vi "Configure RT Noise.vi"(0 "VISA resource name":refnum<visa-resource-name>, 1 "Enable Noise (F:Disable)":bool, 5 "Modulation Format (1: Dual Modulation)":u16(ring)=1 items=["Dual Modulation"=1, "Dual ARB"=2, "Multitone"=3, "Two-tone"=6], 7 "Carrier Bandwidth (1 Hz)":dbl=1.0, 9 "Noise Bandwidth (1 Hz)":dbl=1.0, 11 "error in (no error)":errorcluster, 12 "Noise Bandwidth Factor (1)":u16(ring)=1 items=["1"=1, "2"=2], 13 "Noise Ratio (0 dB)":dbl) -> (4 "VISA resource name out":refnum<visa-resource-name>, 15 "error out":errorcluster)   [LabVIEW 2009, in "Agilent PSG MXG Series.lvlib"]
doc: "Configures real-time additive white gaussian noise (AWGN) added to the carrier.\n\n<B>Notes:</B>\n(1) This VI is valid only in E8267D, N5182A.\n\n(2) For E8267D, this VI is valid only when the instrument installs <B>Option 601</B> or <B>Option 602</B> (Internal baseband generator), and <B>Option 403</B> (Calibrated noise, AWGN).\n\n(3) For N5182A, this VI is valid only when the instrument installs <B>Option 403</B> (Calibrated noise, AWGN)."
uses:
  Agilent PSG MXG Series.lvlib
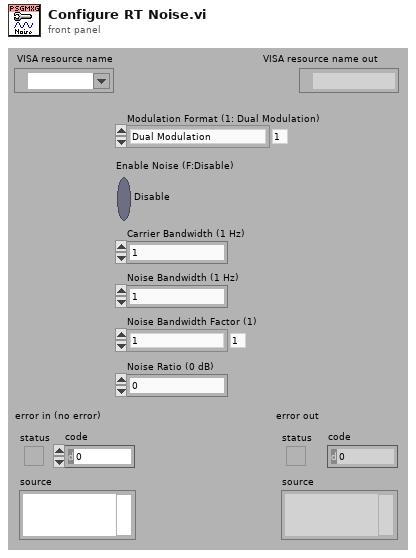
[diagram p1: front panel]
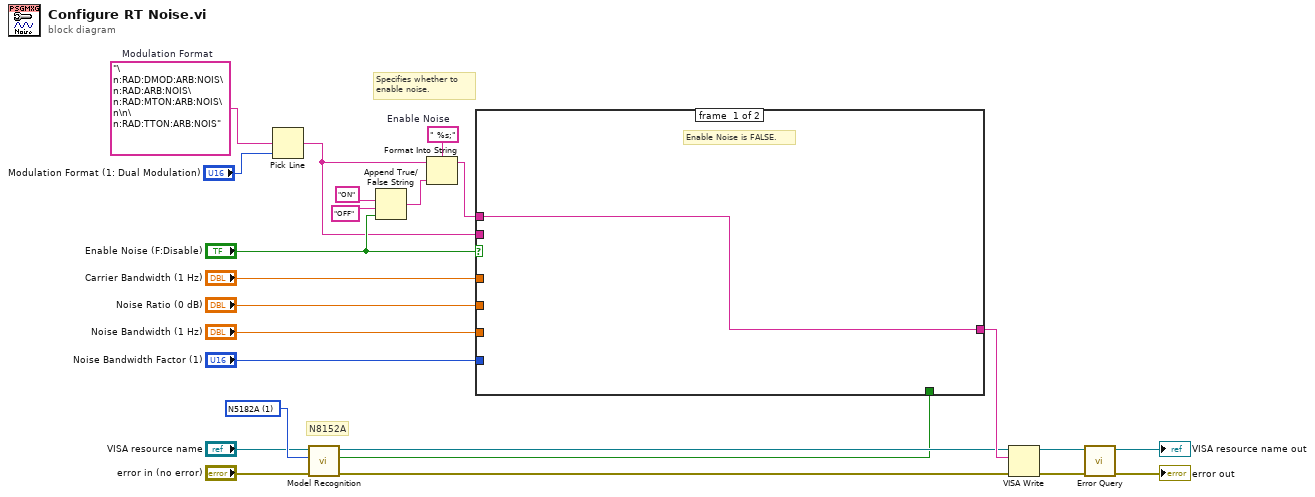
[diagram p0: block diagram]
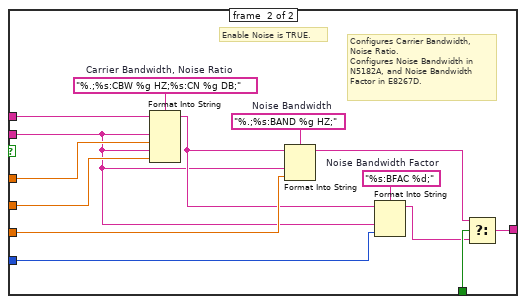
[diagram p2: hidden frame]
diagram:
  w8 = u16 1 items=["N5181A"=0, "N5182A"=1, "E8241A"=5, "E8244A"=6, "E8251A"=7, "E8254A"=8, "E8247C"=10, "E8257C"=11, "E8267C"=12, "E8257D"=15, "E8267D"=16] ("Model Type (0: N5181A)")
  w22 = " %s;"  # Enable Noise
  w24 = "\n:RAD:DMOD:ARB:NOIS\n:RAD:ARB:NOIS\n:RAD:MTON:ARB:NOIS\n\n\n:RAD:TTON:ARB:NOIS"  # Modulation Format
  # "Specifies whether to\nenable noise."
  # "N8152A"
  n1 = Pick Line(multi-line string=w24, line index="Modulation Format (1: Dual Modulation)") -> (output string=w16:string)  [unwired: 1 out]
  n2 = call "Model Recognition.vi"("error in (no error)"="error in (no error)", "Model Type (0: N5181A)"=w8, "VISA resource name"="VISA resource name") -> ("error out"=w6:errorcluster, "Is Model Correct"=w5:bool, "VISA resource name out"=w7:refnum<visa-resource-name>)  [unwired: 6 out]
  n3 = Append True/False String(1:"Enable Noise (F:Disable)", 2:"OFF" ("false string"), 3:"ON" ("true string")) -> (0:w21:string)  [unwired: 1 out]
  n4 = Format Into String(format string=w22, initial string=w16, w21) -> (resulting string=w17:string)  [unwired: 1 in, 1 out]
  n5 = case shown="True" "Enable Noise (F:Disable)" {
    tunnel: w17 -> [w25 w39]
    tunnel: w16 -> [_ w31]
    tunnel: "Carrier Bandwidth (1 Hz)" -> [_ w37]
    tunnel: "Noise Ratio (0 dB)" -> [_ w36]
    tunnel: [w25 w26] -> w9
    tunnel: "Noise Bandwidth (1 Hz)" -> [_ w34]
    tunnel: "Noise Bandwidth Factor (1)" -> [_ w30]
    tunnel: w5 -> [_ w29]
    frame #0 {
      # "Enable Noise is FALSE."
    }
    frame #1 {
      w33 = "%s:BFAC %d;"  # Noise Bandwidth Factor
      w35 = "%.;%s:BAND %g HZ;"  # Noise Bandwidth
      w38 = "%.;%s:CBW %g HZ;%s:CN %g DB;"  # Carrier Bandwidth, Noise Ratio
      # "Configures Carrier Bandwidth,\nNoise Ratio.\nConfigures Noise Bandwidth in\nN5182A, and Noise Bandwidth\nFactor in E8267D."
      # "Enable Noise is TRUE."
      n6 = Format Into String(format string=w38, initial string=w39, w31, w37, w31, w36) -> (resulting string=w32:string)  [unwired: 1 in, 1 out]
      n7 = Format Into String(format string=w35, initial string=w32, w31, w34) -> (resulting string=w28:string)  [unwired: 1 in, 1 out]
      n8 = Format Into String(format string=w33, initial string=w32, w31, w30) -> (resulting string=w27:string)  [unwired: 1 in, 1 out]
      n9 = Select(t=w28, s=w29, f=w27) -> (s? t:f=w26:string)
    }
  }
  n10 = VISA Write(VISA resource name=w7, write buffer=w9, error in (no error)=w6) -> (VISA resource name out=w13:refnum<visa-resource-name>, error out=w12:errorcluster)  [unwired: 1 out]
  n11 = call "Error Query.vi"("error in (no error)"=w12, "VISA resource name"=w13) -> ("error out"=→"error out":errorcluster, "VISA resource name out"=→"VISA resource name out":refnum<visa-resource-name>)  [unwired: 8 out]
